vi "read_from_text_file.vi"(8 "error in (no error)":errorcluster, 10 "file path":path, 11 "PointLinkCollection in":refnum<class "PointLinkCollection.lvclass">) -> (0 "error out":errorcluster, 3 "PointLinkCollection out":refnum<class "PointLinkCollection.lvclass">)   [LabVIEW 2010, in "PointLinkCollection.lvclass"]
uses:
  PointLinkCollection.lvclass
  PointLinkCollection.lvclass/PointLinkCollection.ctl
  <vilib>/Utility/file.llb/Read From Spreadsheet File (DBL).vi
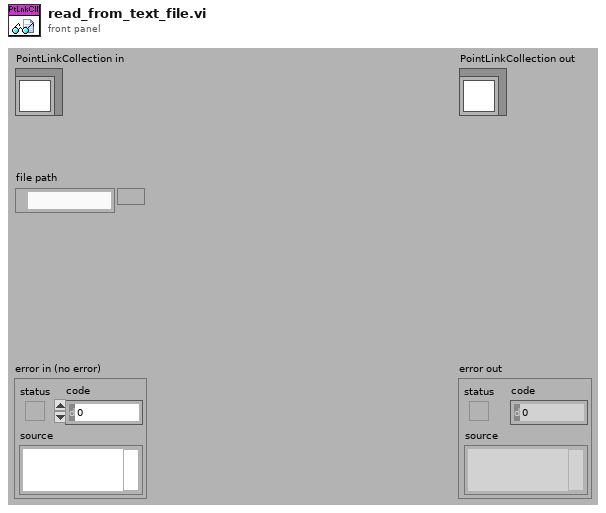
[diagram p1: front panel]
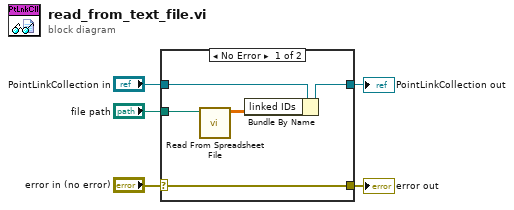
[diagram p0: block diagram]
diagram:
  n1 = case shown="No Error" "error in (no error)" {
    selector: "error in (no error)" -> [w10 w12]
    tunnel: [w10 w12] -> w4
    tunnel: [w6 w11] -> w2
    tunnel: "PointLinkCollection in" -> [w7 w11]
    tunnel: "file path" -> [w9 _]
    frame No Error {
      n2 = call-poly <vilib>:"Read From Spreadsheet File.vi"("file path (dialog if empty)"=w9) -> ("all rows"=w8:dbl[][])  [unwired: 6 in, 4 out]
      n3 = Bundle By Name(cluster=w7, "linked IDs"=w8) -> (w6:refnum<class "PointLinkCollection.lvclass">)
    }
    frame Error {
    }
  }
  "error out" <- w4
  "PointLinkCollection out" <- w2
